vi "manualGain.vi"(10 "Use DDS display equivalent?":bool, 11 "Gain (arb)":i16) -> (2 "DDS display value":i16, 3 "Photodiode string out":string)   [LabVIEW 2012, in "DDS9954_v2013.lvlib"]
uses:
  DDS9954_v2013.lvlib
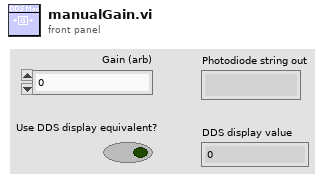
[diagram p1: front panel]
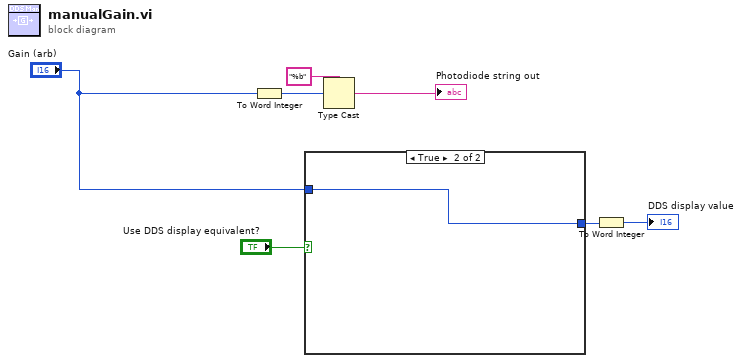
[diagram p0: block diagram]
diagram:
  n1 = To Word Integer(number="Gain (arb)") -> (16bit integer=w7:i16)
  n2 = case shown="True" "Use DDS display equivalent?" {
    tunnel: "Gain (arb)" -> [w8 w9]
    tunnel: [w8 w9] -> w3
    frame False {
    }
    frame True {
    }
  }
  n3 = Type Cast(type="%b", x=w7) -> (*(type *) &x=→"Photodiode string out":string)
  n4 = To Word Integer(number=w3) -> (16bit integer=→"DDS display value":i16)
